vi "Delete Elements from 2D Array (EXT)__ogtk.vi"(8 "delete (rows or columns)":enum16{"rows", "columns"}(ring), 9 "indices":i32[](array[numeric]), 11 "array":ext[][](array[numeric]) format="%.2f") -> (1 "deleted elements":ext[][](array[numeric]) format="%.2f", 3 "array w/ subset deleted":ext[][](array[numeric]) format="%.2f")   [LabVIEW 2014]
doc: "This polymorphic VI deletes elements from a 1D or 2D <B>array</B> at the corresponding <B>indices</B>, returning <B>array w/ subset deleted</B> and <B>deleted elements</B>. For 2D arrays, wire the <B>delete (rows or columns)</B> input to specify whether to delete rows or columns."
uses:
  <userlib>/_OpenG.lib/array/array.llb/Sort 1D Array (I32)__ogtk.vi
  <userlib>/_OpenG.lib/array/array.llb/Reorder 2D Array2 (EXT)__ogtk.vi
panel:
  # "Delete Elements from Array.vi\n\nThis polymorphic VI deletes elements from a 1D or 2D array at the corresponding indices\n\nPlease visit http://www.OpenG.org to learn about the\nOpen Source LabVIEW software movement.\n\nNOTICE -- YOU MUST LEAVE THIS NOTICE IN PLACE.  PER THE TERMS OF THE LICENSE BELOW, YOU MAY SUBLICENSE THIS SOFTWARE \nIN ANY WAY THAT DOES NOT CONFLICT WITH THIS LICENSE.\n\n### BSD License (http://www.opensource.org/licenses/bsd-license.php) Begin ###\n \nCopyright (c) 2007, JKI <info@jameskring.com> \nCopyright (c) 2007, Jim Kring <jim.kring@jameskring.com>\nCopyright (c) 2011, Jonathon Green <jg@jgcode.net>\n\nAll rights reserved.\n\nRedistribution and use in source and binary forms, with or without modification, are permitted provided that the following conditions are met:\n\n    * Redistributions of source code must retain the above copyright notice, this list of conditions and the following disclaimer.\n    * Redistributions in binary form must reproduce the above copyright notice, this list of conditions and the following disclaimer in the \n       documentation and/or other materials provided with the distribution.\n    * Neither the name of SciWare, James Kring, Inc., nor the names of its contributors may be used to endorse or promote products derived \n       from this software without specific prior written permission.\n\nTHIS SOFTWARE IS PROVIDED BY THE COPYRIGHT HOLDERS AND CONTRIBUTORS \"AS IS\" AND ANY EXPRESS OR IMPLIED WARRANTIES, \nINCLUDING, BUT NOT LIMITED TO, THE IMPLIED WARRANTIES OF MERCHANTABILITY AND FITNESS FOR A PARTICULAR PURPOSE ARE \nDISCLAIMED. IN NO EVENT SHALL THE COPYRIGHT OWNER OR CONTRIBUTORS BE LIABLE FOR ANY DIRECT, INDIRECT, INCIDENTAL,\n SPECIAL, EXEMPLARY, OR CONSEQUENTIAL DAMAGES (INCLUDING, BUT NOT LIMITED TO, PROCUREMENT OF SUBSTITUTE GOODS OR \nSERVICES; LOSS OF USE, DATA, OR PROFITS; OR BUSINESS INTERRUPTION) HOWEVER CAUSED AND ON ANY THEORY OF LIABILITY, \nWHETHER IN CONTRACT, STRICT LIABILITY, OR TORT (INCLUDING NEGLIGENCE OR OTHERWISE) ARISING IN ANY WAY OUT OF THE USE \nOF THIS SOFTWARE, EVEN IF ADVISED OF THE POSSIBILITY OF SUCH DAMAGE.\n\n### BSD License End ###"
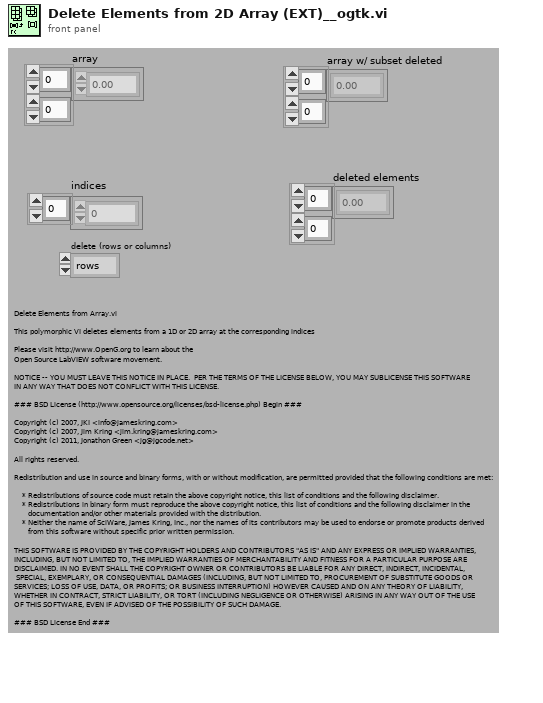
[diagram p1: front panel]
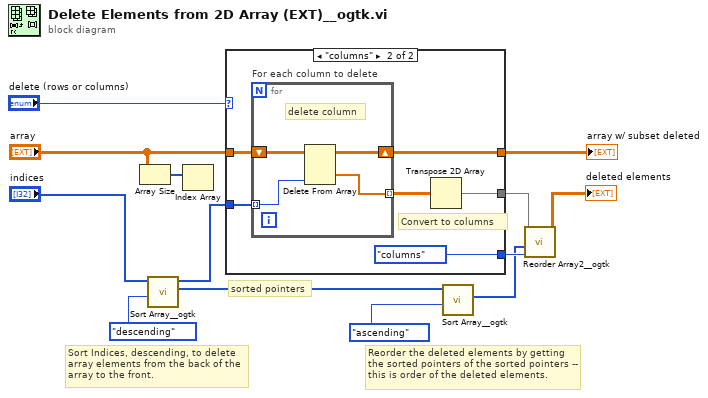
[diagram p0: block diagram]
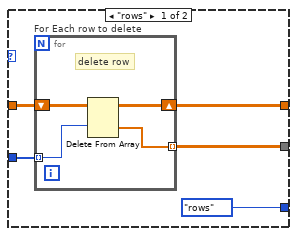
[diagram p2: hidden frame]
diagram:
  # "Reorder the deleted elements by getting the sorted pointers of the sorted pointers -- this is order of the deleted elements."
  # "Sort Indices, descending, to delete array elements from the back of the array to the front."
  # "sorted pointers"
  n1 = Array Size(array="array") -> (size(s)=w5:i32[])
  n2 = call-poly <userlib>:"Sort Array__ogtk.vi"("Order"=enum16{"ascending", "descending"}."descending", "Array in"="indices") -> ("Sorted Pointers"=w9:i32[], "Sorted Array out"=w8:i32[])  [unwired: 8 in]
  n3 = Index Array(array=w5) -> ()  [unwired: 1 in, 1 out]
  n4 = case shown="\"columns\"" "delete (rows or columns)" {
    tunnel: [w18 w28] -> w13
    tunnel: w8 -> [w17 w27]
    tunnel: "array" -> [w16 w26]
    tunnel: [w15 w24] -> w4
    tunnel: [enum16{"rows", "columns"}."rows" ("reorder (rows)") enum16{"rows", "columns"}."columns" ("reorder (rows)")] -> w2
    frame "rows" {
      n5 = for "For Each row to delete" {
        tunnel: w17 -> [w22] mode=indexing
        shift-right: [w21] -> w18
        shift-left: w16 -> [w20]
        tunnel: [w19] -> w15 mode=indexing
        # "delete row"
        n6 = Delete From Array(array=w20, index (row)=w22) -> (deleted portion=w19:ext[], array with subset deleted=w21:ext[][])  [unwired: 2 in]
      }
    }
    frame "columns" {
      # "Convert to columns"
      n7 = for "For each column to delete" {
        tunnel: w27 -> [w29] mode=indexing
        shift-right: [w32] -> w28
        shift-left: w26 -> [w31]
        tunnel: [w30] -> w25 mode=indexing
        # "delete column"
        n8 = Delete From Array(array=w31, index (col)=w29) -> (deleted portion=w30:ext[], array with subset deleted=w32:ext[][])  [unwired: 2 in]
      }
      n9 = Transpose 2D Array(2D array=w25) -> (transposed array=w24:ext[][])
    }
  }
  "array w/ subset deleted" <- w13
  n10 = call-poly <userlib>:"Sort Array__ogtk.vi"("Order"=enum16{"ascending", "descending"}."ascending", "Array in"=w9) -> ("Sorted Pointers"=w1:i32[])  [unwired: 8 in, 1 out]
  n11 = call-poly <userlib>:"Reorder Array2__ogtk.vi"("reorder (rows)"=w2, "indices"=w1, "array"=w4) -> ("reordered array"=→"deleted elements":ext[][])  [unwired: 8 in]
